vi "BoxDouble.vi"(10 "Numeric":dbl) -> (2 "Double out":refnum<class "Double.lvclass">)   [LabVIEW 2013, in "LapDog.Collections.v_.Common.lvlib" / "Double.lvclass"]
uses:
  Double.lvclass
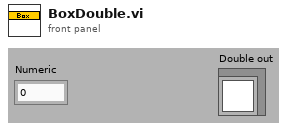
[diagram p1: front panel]
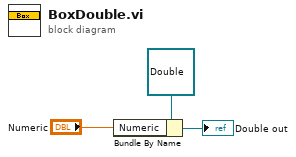
[diagram p0: block diagram]
diagram:
  n1 = Bundle By Name(cluster=refnum<class "Double.lvclass"> refnum ("LapDog.Collections.v0.Lists.Interfaces.lvlib:String.lvclass"), "Numeric"="Numeric") -> (→"Double out":refnum<class "Double.lvclass">)
